vi "OpenCamera.vi"(0 "object in":refnum<class "Hamamatsu.lvclass">, 5 "error in (no error)":errorcluster) -> (14 "object out":refnum<class "Hamamatsu.lvclass">, 16 "CameraConnected":bool, 19 "error out":errorcluster)   [LabVIEW 2019, in "Hamamatsu.lvclass"]
uses:
  Hamamatsu.lvclass
  Hamamatsu.lvclass/Hamamatsu.ctl
panel:
  out "Camera Details":T1
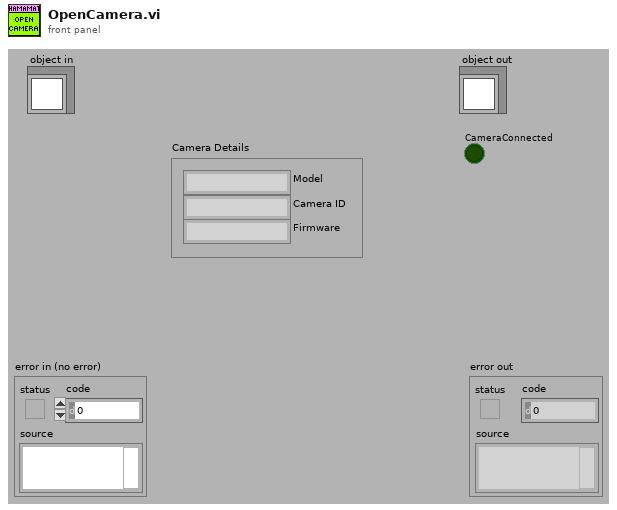
[diagram p1: front panel]
types:
  T1 = cluster{"Model":string, "Camera ID":string, "Firmware":string}
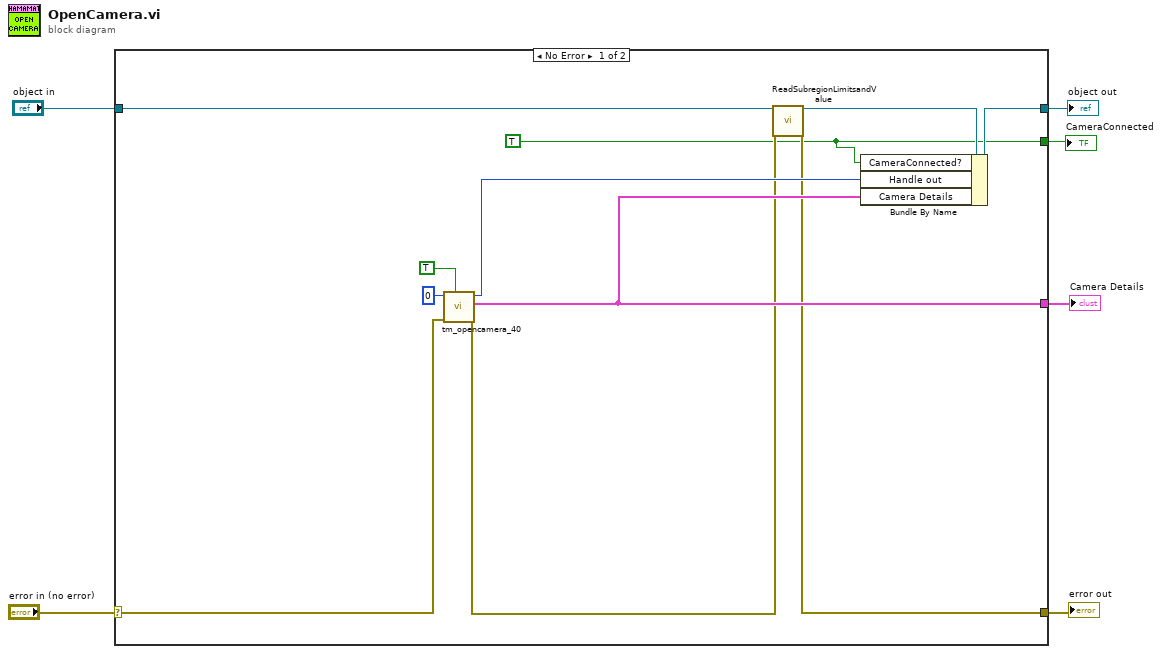
[diagram p0: block diagram]
diagram:
  n1 = case shown="No Error" "error in (no error)" {
    selector: "error in (no error)" -> [w14 w19]
    tunnel: [w10 w19] -> w5
    tunnel: [w16 w18] -> w3
    tunnel: "object in" -> [w11 w18]
    tunnel: [w15 _] -> w2
    tunnel: [w7 _] -> w1
    frame No Error {
      w7 = TRUE ("CameraConnected")
      n2 = call <userlib>:"tm_opencamera_40.vi"("Force Open"=TRUE, "error in (no error)"=w14, "Camera Index"=u32 0) -> ("error out"=w12:errorcluster, "Camera Details"=w15:T1, "Handle out"=w13:u32)  [unwired: 6 in]
      n3 = call-dynamic "ReadSubregionLimitsandValue.vi"("object in"=w11, "error in (no error)"=w12) -> ("object out"=w9:refnum<class "Hamamatsu.lvclass">, "error out"=w10:errorcluster)  [unwired: 15 in, 1 out]
      n4 = Bundle By Name(cluster=w9, "CameraConnected?"=w7, "Handle out"=w13, "Camera Details"=w15) -> (w16:refnum<class "Hamamatsu.lvclass">)
    }
    frame Error {
    }
  }
  "error out" <- w5
  "object out" <- w3
  "Camera Details" <- w2
  "CameraConnected" <- w1
